vi "Network Write.vi"(7 "Values":dbl[](array[numeric]), 8 "error in (no error)":errorcluster, 9 "Status_Cluster":T1={"simTime"=0.0, "simFrame"=0.0, "Connection Status"=enum."Disconnected", "Connection Command"=enum."Disconnect", "Last Error"=0, "Case selection"=enum."Connecting"}, 10 "RDB References in":T7, 11 "Settings in":T4={"UDP Receiver"=refnum, "UDP Sender"=refnum, "Valid Packet"=FALSE, "TCP"=refnum, "Network Settings"={"IP adress"="127.0.0.1", "RDB"={"Protocol"=enum."UDP", "Tx Port"=48270, "Rx Port"=10, "Buffer Size"=204800, "Timeout"=10}, "SCP"={"Protocol"=enum."TCP", "Tx Port"=48191, "Rx Port"=48191, "Buffer Size"=204800, "Timeout"=10}}, "vclient"=path "", "paeseHandle"=0, "builderHandle"=0}) -> (0 "error out":errorcluster, 2 "RDB Reference out":T7, 3 "Settings out":T4={"UDP Receiver"=refnum, "UDP Sender"=refnum, "Valid Packet"=FALSE, "TCP"=refnum, "Network Settings"={"IP adress"="127.0.0.1", "RDB"={"Protocol"=enum."UDP", "Tx Port"=48270, "Rx Port"=10, "Buffer Size"=204800, "Timeout"=10}, "SCP"={"Protocol"=enum."TCP", "Tx Port"=48191, "Rx Port"=48191, "Buffer Size"=204800, "Timeout"=10}}, "vclient"=path "", "paeseHandle"=0, "builderHandle"=0})   [LabVIEW 2023, in "Vires VTD Engine.lvlib"]
uses:
  Vires VTD Engine.lvlib
  RDB/RDB References.ctl
  DataContainer/DataContainer.lvclass
  Type/Settings.ctl
  Shared/Network Settings.ctl
  Shared/Protocol.ctl
  Type/Status_Cluster.ctl
  Type/ConnectionStatus.ctl
  Type/CaseSelection.ctl
  RDB/RDB.lvlib
  Shared/Vires VTD Shared.lvlib
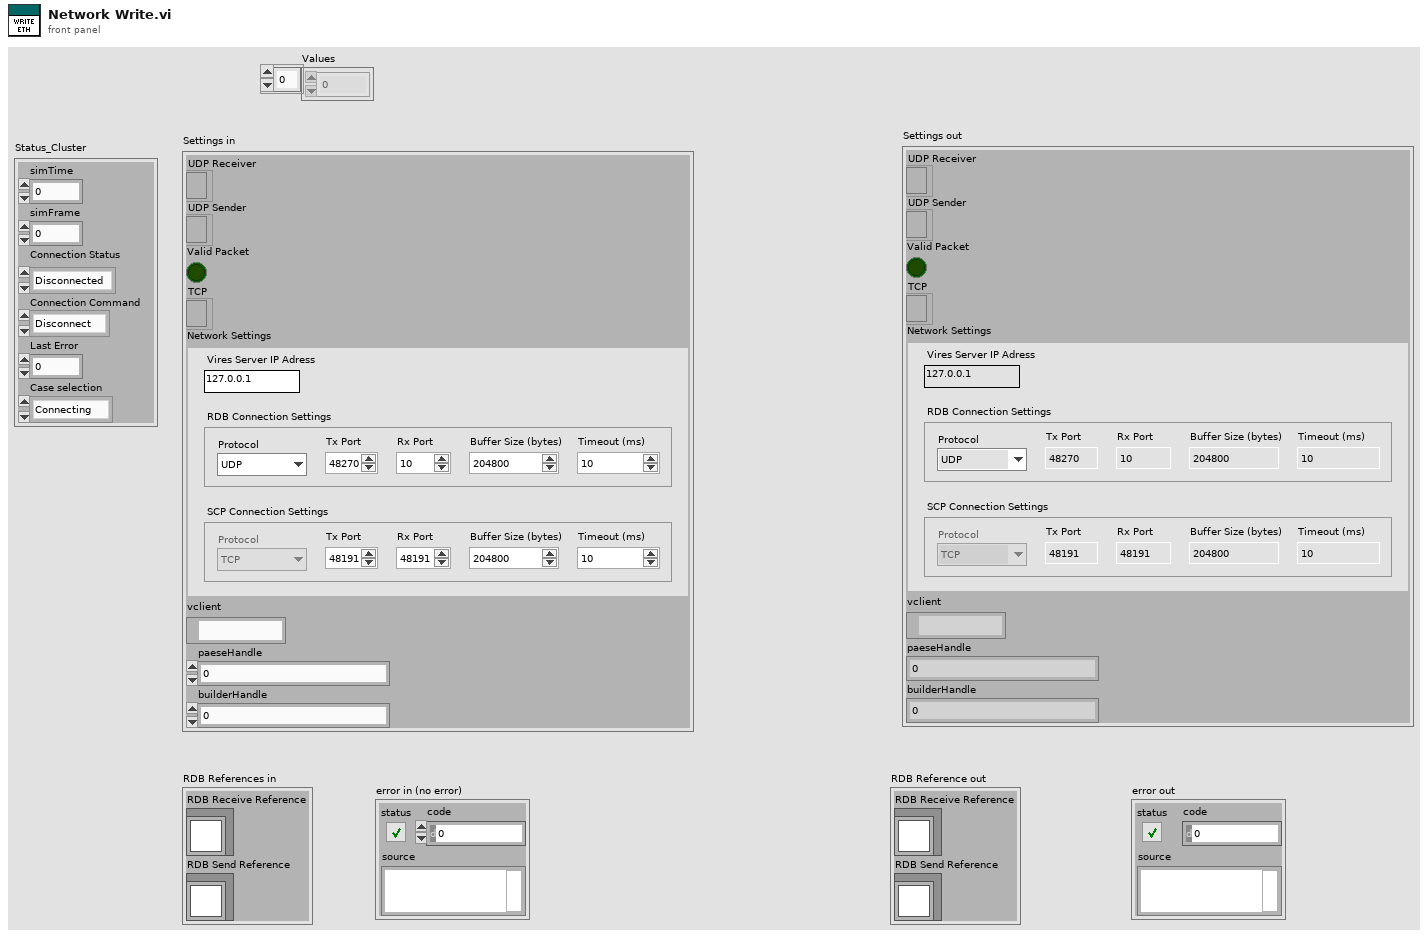
[diagram p1: front panel]
types:
  T1 = typedef "Vires VTD Engine.lvlib/Status_Cluster.ctl" = cluster{"simTime":dbl, "simFrame":dbl, "Connection Status":T2, "Connection Command":enum16{"Disconnect", "Connect"}, "Last Error":i32, "Case selection":T3}
  T2 = typedef "Vires VTD Engine.lvlib/ConnectionStatus.ctl" = enum16{"Disconnected", "Connected"}
  T3 = typedef "Vires VTD Engine.lvlib/CaseSelection.ctl" = enum32{"Idle", "Connecting", "Disconnecting", "Read/Write"}
  T4 = typedef "Vires VTD Engine.lvlib/Settings.ctl" = cluster{"UDP Receiver":refnum<k16>, "UDP Sender":refnum<k16>, "Valid Packet":bool, "TCP":refnum<k5>, "Network Settings":T5, "vclient":path, "paeseHandle":u64, "builderHandle":u64}
  T5 = typedef "Vires VTD Shared.lvlib/Network Settings.ctl" = cluster{"IP adress":string, "RDB":cluster{"Protocol":T6, "Tx Port":u16, "Rx Port":u16, "Buffer Size":i32, "Timeout":u16}, "SCP":cluster{"Protocol":T6, "Tx Port":u16, "Rx Port":u16, "Buffer Size":i32, "Timeout":u16}}
  T6 = typedef "Vires VTD Shared.lvlib/Protocol.ctl" = enum16{"UDP", "TCP"}
  T7 = typedef "RDB.lvlib/RDB References.ctl" = cluster{"RDB Receive Reference":refnum<class "DataContainer.lvclass">, "RDB Send Reference":refnum<class "DataContainer.lvclass">}
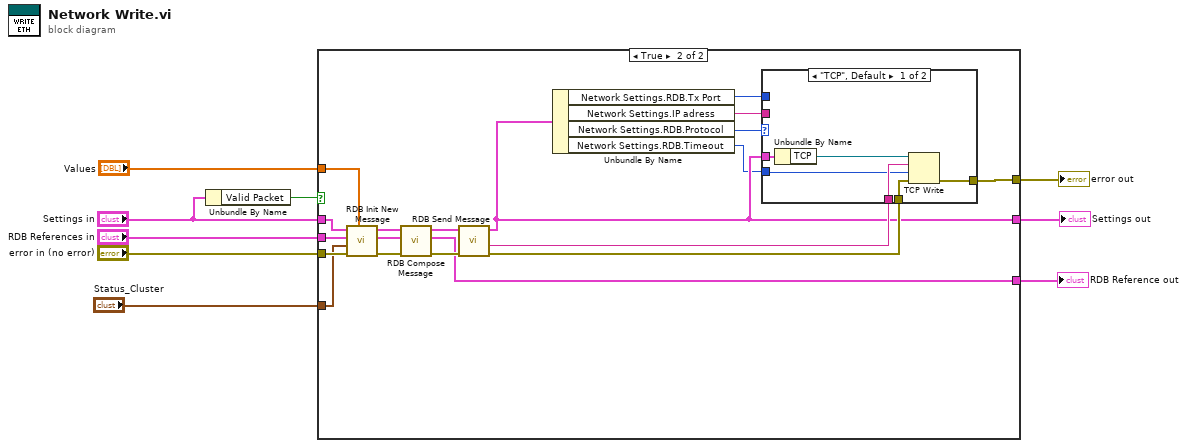
[diagram p0: block diagram]
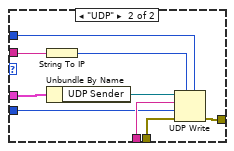
[diagram p3: hidden frame]
diagram:
  n1 = Unbundle By Name("Settings in") -> ("Valid Packet"=w5:bool)
  n2 = case shown="True" w5 {
    tunnel: [w12 w30] -> w9
    tunnel: [w11 w13] -> w8
    tunnel: "error in (no error)" -> [w12 w25]
    tunnel: "Values" -> [_ w24]
    tunnel: "RDB References in" -> [w11 w18]
    tunnel: "Settings in" -> [w10 w17]
    tunnel: [w10 w16] -> w2
    tunnel: "Status_Cluster" -> [_ w14]
    frame False {
    }
    frame True {
      n3 = call "RDB Init New Message.vi"("RDB Receive Reference.RDB Signals"=w24, "error in (no error)"=w25, "Status_Cluster"=w14, "RDB Reference in"=w18, "Settings in"=w17) -> ("error out"=w26:errorcluster, "RDB Reference out"=w19:T7, "Settings out"=w31:T4)  [unwired: 4 in]
      n4 = call "RDB Compose Message.vi"("error in (no error)"=w26, "RDB Reference in"=w19, "Settings in"=w31) -> ("error out"=w27:errorcluster, "RDB Reference out"=w13:T7, "Settings out"=w28:T4)  [unwired: 6 in]
      n5 = call "RDB Send Message.vi"("error in (no error)"=w27, "Settings in"=w28) -> ("error out"=w29:errorcluster, "RDB Message"=w20:string, "Settings out"=w16:T4)  [unwired: 7 in]
      n6 = Unbundle By Name(w16) -> ("Network Settings.RDB.Tx Port"=w21:u16, "Network Settings.IP adress"=w22:string, "Network Settings.RDB.Protocol"=w23:T6, "Network Settings.RDB.Timeout"=w15:u16)
      n7 = case shown="\"TCP\", Default" w23 {
        tunnel: w20 -> [w33 w45]
        tunnel: [w34 w44] -> w30
        tunnel: w29 -> [w35 w43]
        tunnel: w16 -> [w37 w41]
        tunnel: w22 -> [_ w40]
        tunnel: w21 -> [_ w39]
        tunnel: w15 -> [w32 w38]
        frame "TCP", Default {
          n8 = Unbundle By Name(w37) -> ("TCP"=w36:refnum<k5>)
          n9 = TCP Write(connection ID=w36, data in=w33, error in (no error)=w35, 9:w32) -> (error out=w34:errorcluster)  [unwired: 2 out]
        }
        frame "UDP" {
          n10 = String To IP(1:w40) -> (0:w46:u32)
          n11 = Unbundle By Name(w41) -> ("UDP Sender"=w42:refnum<k16>)
          n12 = UDP Write(address=w46, port or service name=w39, connection ID=w42, data in=w45, 8:w43, 9:w38) -> (error out=w44:errorcluster)  [unwired: 1 out]
        }
      }
    }
  }
  "error out" <- w9
  "RDB Reference out" <- w8
  "Settings out" <- w2
